vi "FTW-TransferClient-Construct.vi"(0 "Access Key":string, 1 "Region":string, 5 "Secret Key":string, 7 "Bucket":string, 9 "Subfolder":string, 11 "error in":errorcluster, 12 "Headers":T1[](array[typedef])) -> (4 "Transfer Client":refnum<class "FTW-TransferClient-S3.lvclass">, 15 "error out":errorcluster)   [LabVIEW 2014, in "FTW-TransferClient-S3.lvclass"]
uses:
  FTW-TransferClient-S3.lvclass
  sandbox/deprecated/FTW-Collection-KeyValuePair.ctl
  C:/Users/Jack/repo/ftw-master/ftw/src/windows/transfer/S3/AWSSDK.dll
  AWSSDK.dll
  FTW-TransferClient-S3.lvclass/FTW-TransferClient-S3.ctl
panel:
  # "Inputs"
  # "Outputs"
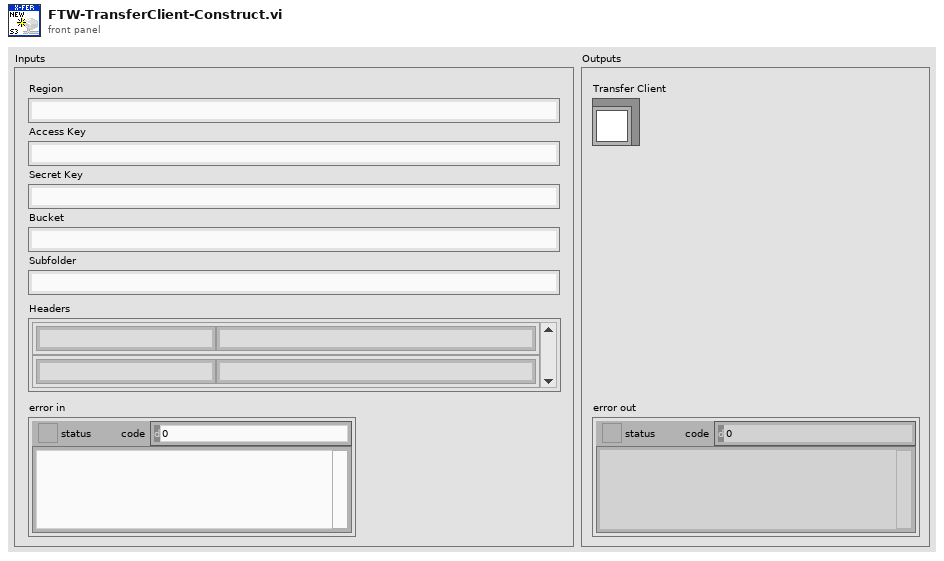
[diagram p1: front panel]
types:
  T1 = typedef "FTW-Collection-KeyValuePair.ctl" = cluster{"Key":string, "Value":string}
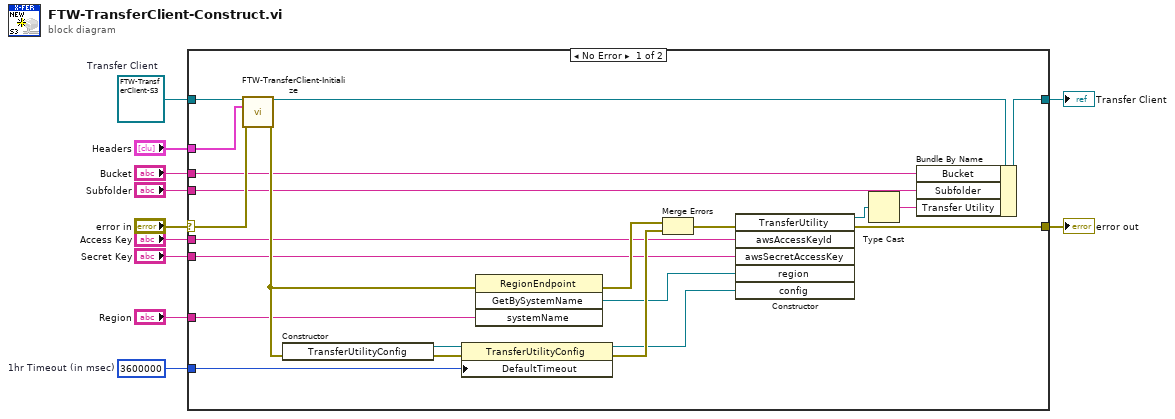
[diagram p0: block diagram]
diagram:
  w8 = refnum<class "FTW-TransferClient-S3.lvclass"> refnum  # Transfer Client
  w9 = 3600000  # 1hr Timeout (in msec)
  n1 = case shown="No Error" "error in" {
    selector: "error in" -> [w18 w34]
    tunnel: w8 -> [w21 w35]
    tunnel: [w33 w35] -> w11
    tunnel: [w32 w34] -> w10
    tunnel: w9 -> [w25 _]
    tunnel: "Headers" -> [w19 _]
    tunnel: "Region" -> [w16 _]
    tunnel: "Secret Key" -> [w15 _]
    tunnel: "Access Key" -> [w14 _]
    tunnel: "Bucket" -> [w13 _]
    tunnel: "Subfolder" -> [w12 _]
    frame No Error {
      n2 = call-dynamic "FTW-TransferClient-Initialize.vi"("Transfer Client"=w21, "Headers"=w19, "error in"=w18) -> ("Transfer Client out"=w20:refnum<class "FTW-TransferClient-S3.lvclass">, "error out"=w17:errorcluster)  [unwired: 11 in]
      n3 = constructor class="TransferUtilityConfig"(error in=w17) -> (reference out=w29:refnum<k24>, error out=w28:errorcluster)  [unwired: 2 in, 1 out]
      n4 = property class="TransferUtilityConfig"(reference=w29, error in=w28, "DefaultTimeout"=w25) -> (reference out=w24:refnum<k24>, error out=w26:errorcluster)
      n5 = invoke class="RegionEndpoint" method="GetBySystemName"(error in=w17, "systemName"=w16) -> (error out=w23:errorcluster, "GetBySystemName"=w22:refnum<k24>)  [unwired: 2 in, 2 out]
      n6 = Merge Errors(w23, w26) -> (w27:errorcluster)
      n7 = constructor class="TransferUtility"(error in=w27, "awsAccessKeyId"=w14, "awsSecretAccessKey"=w15, "region"=w22, "config"=w24) -> (reference out=w31:refnum<k24>, error out=w32:errorcluster)  [unwired: 2 in, 5 out]
      n8 = Type Cast(x=w31) -> (*(type *) &x=w30:string)  [unwired: 1 in]
      n9 = Bundle By Name(cluster=w20, "Bucket"=w13, "Subfolder"=w12, "Transfer Utility"=w30) -> (w33:refnum<class "FTW-TransferClient-S3.lvclass">)
    }
    frame Error {
    }
  }
  "error out" <- w10
  "Transfer Client" <- w11
